vi "Obtain Result.vi"(8 "Error In":errorcluster, 9 "Default Result":refnum<class "IResult.lvclass">, 10 "Name":string, 11 "Logger In":refnum<class "LoggerAPI.lvclass">) -> (0 "Error Out":errorcluster, 1 "Result Out":refnum<class "IResult.lvclass">, 2 "Result Not Found?":bool, 3 "Logger Out":refnum<class "LoggerAPI.lvclass">)   [LabVIEW 2019, in "LoggerAPI.lvclass"]
uses:
  LoggerAPI.lvclass
  IResult/IResult.lvclass
  LoggerAPI.lvclass/LoggerAPI.ctl
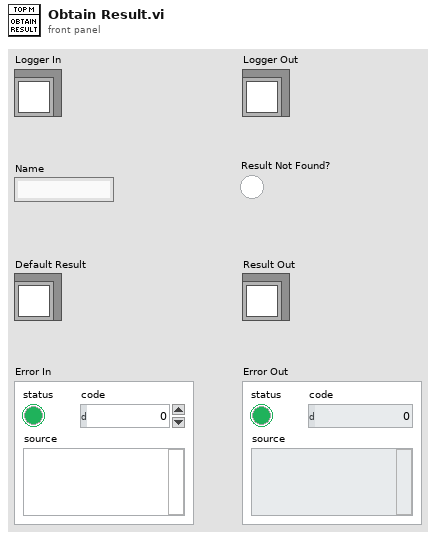
[diagram p1: front panel]
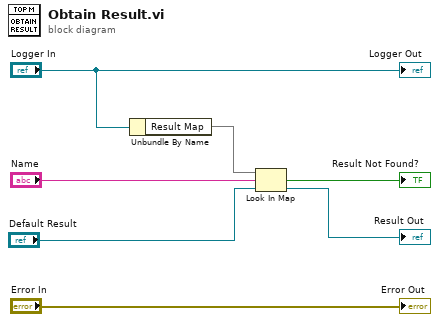
[diagram p0: block diagram]
diagram:
  n1 = Unbundle By Name("Logger In") -> ("Result Map"=w6:map{string, refnum<class "IResult.lvclass">})
  n2 = Look In Map(map=w6, key="Name", default value="Default Result") -> (key not found?=→"Result Not Found?":bool, value=→"Result Out":refnum<class "IResult.lvclass">)
  "Logger Out" <- "Logger In"
  "Error Out" <- "Error In"
